vi "用户信息.vi"(2 "口令":string, 3 "用户名":string) -> (0 "访问确认":bool, 1 "访问权限":string)   [LabVIEW 2010]
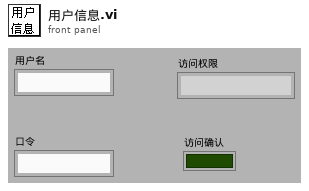
[diagram p1: front panel]
types:
  T1 = cluster{"用户名":string, "口令":string, "访问权限":string}[]
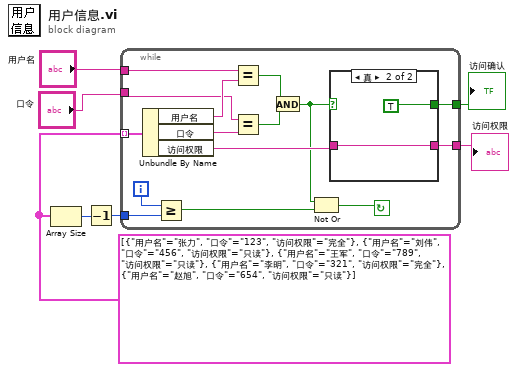
[diagram p0: block diagram]
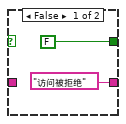
[diagram p2: hidden frame]
diagram:
  w4 = T1 [{"用户名"="张力", "口令"="123", "访问权限"="完全"}, {"用户名"="刘伟", "口令"="456", "访问权限"="只读"}, {"用户名"="王军", "口令"="789", "访问权限"="只读"}, {"用户名"="李明", "口令"="321", "访问权限"="完全"}, {"用户名"="赵旭", "口令"="654", "访问权限"="只读"}]
  n1 = Array Size(array=w4) -> (size(s)=w2:i32)
  n2 = Decrement(x=w2) -> (x-1=w1:i32)
  n3 = while {
    tunnel: w4 -> [w22] mode=indexing
    tunnel: "用户名" -> [w19]
    tunnel: "口令" -> [w17]
    tunnel: [w14] -> w5
    tunnel: w1 -> [w12]
    tunnel: [w8] -> w3
    i -> [w13]
    stop <- w11 continue-if-true
    n4 = Unbundle By Name(w22) -> ("用户名"=w18:string, "口令"=w16:string, "访问权限"=w15:string)
    n5 = Greater Or Equal?(x=w13, y=w12) -> (x >= y?=w9:bool)
    n6 = Equal?(x=w19, y=w18) -> (x = y?=w21:bool)
    n7 = Equal?(x=w17, y=w16) -> (x = y?=w20:bool)
    n8 = And(x=w21, y=w20) -> (x .and. y?=w10:bool)
    n9 = Not Or(1:w9, 2:w10) -> (0:w11:bool)
    n10 = case shown="真" w10 {
      tunnel: w15 -> [_ w26]
      tunnel: ["访问被拒绝" w26] -> w14
      tunnel: [FALSE TRUE] -> w8
      frame False {
      }
      frame True {
      }
    }
  }
  "访问权限" <- w5
  "访问确认" <- w3
